vi "ParseIdentifierResponse.vi"(8 "error in (no error)":errorcluster, 11 "Value":string) -> (0 "error out":errorcluster, 2 "status":string, 3 "description":string)   [LabVIEW 2021]
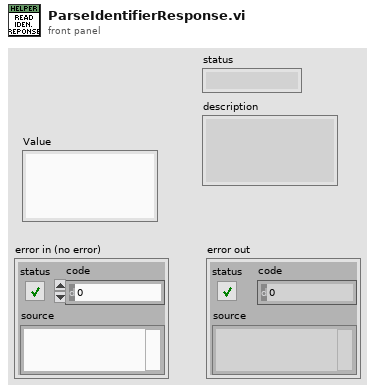
[diagram p1: front panel]
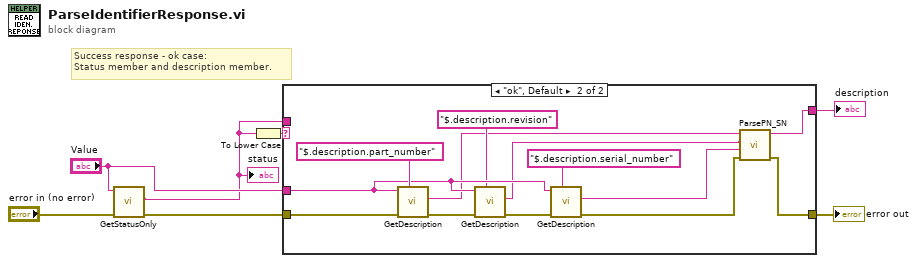
[diagram p0: block diagram]
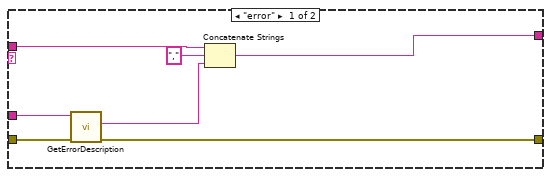
[diagram p2: hidden frame]
diagram:
  # "Success response - ok case:\nStatus member and description member."
  n1 = call "GetStatusOnly.vi"("error in (no error)"="error in (no error)", "Value"="Value") -> ("error out"=w5:errorcluster, "status"=w2:string)  [unwired: 7 in, 1 out]
  "status" <- w2
  n2 = To Lower Case(string=w2) -> (all lower case string=w3:string)
  n3 = case shown="\"ok\", Default" w3 {
    tunnel: [w12 w16] -> w4
    tunnel: "Value" -> [w14 w23]
    tunnel: w5 -> [w13 w27]
    tunnel: [w9 w15] -> w1
    tunnel: w2 -> [w8 _]
    frame "error" {
      n4 = call "GetErrorDescription.vi"("error in (no error)"=w13, "Value"=w14) -> ("error out"=w12:errorcluster, "description"=w10:string)  [unwired: 7 in, 1 out]
      n5 = Concatenate Strings(w8, "," ("string"), w10) -> (w9:string)
    }
    frame "ok", Default {
      n6 = call "GetDescription.vi"("$Path or Item Name"="$.description.part_number", "error in (no error)"=w27, "Value"=w23) -> ("error out"=w25:errorcluster, "description"=w18:string)  [unwired: 7 in]
      n7 = call "GetDescription.vi"("$Path or Item Name"="$.description.revision", "error in (no error)"=w25, "Value"=w23) -> ("error out"=w24:errorcluster, "description"=w19:string)  [unwired: 7 in]
      n8 = call "GetDescription.vi"("$Path or Item Name"="$.description.serial_number", "error in (no error)"=w24, "Value"=w23) -> ("error out"=w17:errorcluster, "description"=w20:string)  [unwired: 7 in]
      n9 = call "ParsePN_SN.vi"("error in (no error)"=w17, "SerialNumber"=w20, "Revision"=w19, "PartNumber"=w18) -> ("error out"=w16:errorcluster, "description"=w15:string)  [unwired: 6 in]
    }
  }
  "error out" <- w4
  "description" <- w1
